vi "Test Preview Element.vi"() -> ()   [LabVIEW 2013]
uses:
  <vilib>/addons/_JKI Toolkits/Caraya/classes/Assert/Assert True.vi
  Circular Buffers/ByteFIFO/ByteFIFO.lvclass
  Circular Buffers/VariantBuffer/VariantBuffer.lvclass
  <vilib>/addons/_JKI Toolkits/Caraya/classes/Test/Test.lvclass
  <vilib>/addons/_JKI Toolkits/Caraya/classes/Assert/Assert.lvclass
panel:
  out "bytes 3":u8[](array[numeric]) format="%02x"
  out "bytes 2":u8[](array[numeric]) format="%02x"
  out "bytes":u8[](array[numeric]) format="%02x"
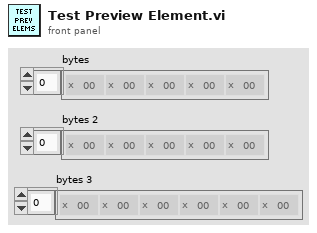
[diagram p1: front panel]
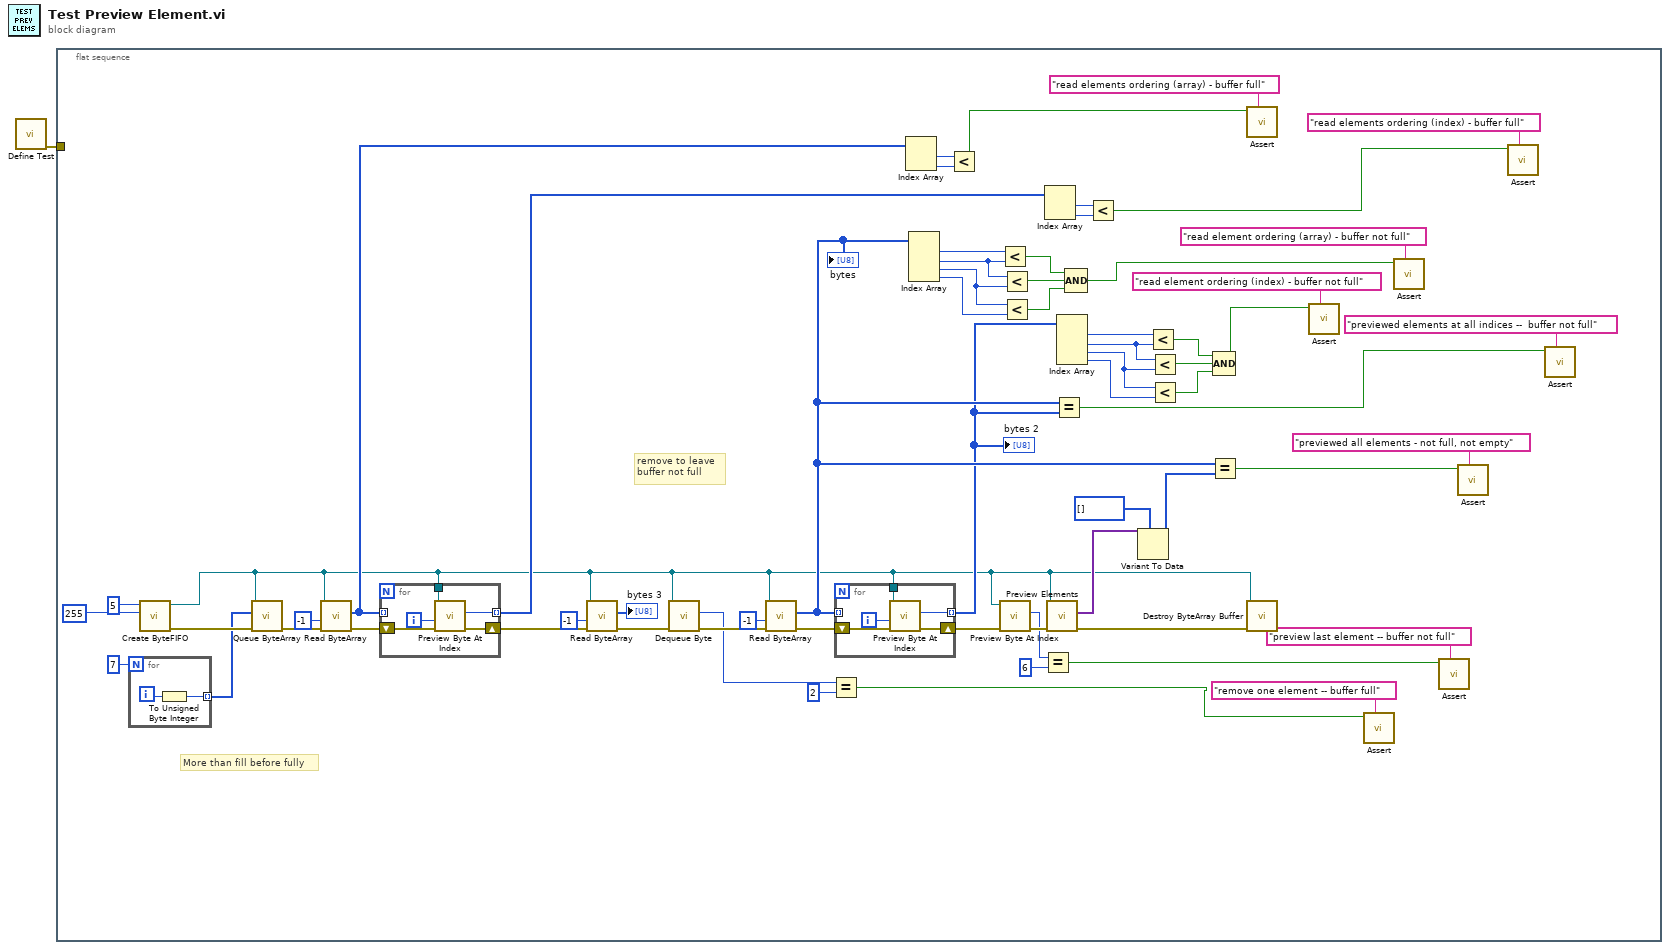
[diagram p0: block diagram]
diagram:
  n1 = call <vilib>:"Define Test.vi"() -> ("error out"=w1:errorcluster)  [unwired: 10 in, 1 out]
  n2 = flat-sequence {
    tunnel: w1 -> [_]
    frame #0 {
      # "remove to leave \nbuffer not full"
      # "More than fill before fully"
      n3 = for {
        N: 7 -> [_]
        tunnel: [w76] -> w61 mode=indexing
        i -> [w77]
        n4 = To Unsigned Byte Integer(number=w77) -> (unsigned 8bit integer=w76:u8)
      }
      n5 = call "Create ByteFIFO.vi"("default value"=u8 255, "bufSize"=5) -> ("error out"=w63:errorcluster, "Buffer"=w22:refnum<data-value>)  [unwired: 8 in]
      n6 = call "Queue ByteArray.vi"("error in"=w63, "bytes"=w61, "Buffer"=w22) -> ("error out"=w50:errorcluster)  [unwired: 6 in, 2 out]
      n7 = call "Read ByteArray.vi"("error in"=w50, "count (-1: all)"=-1, "Buffer"=w22) -> ("error out"=w47:errorcluster, "bytes"=w46:u8[])  [unwired: 6 in, 1 out]
      n8 = for {
        tunnel: w22 -> [w68]
        tunnel: [w67] -> w43 mode=indexing
        shift-right: [w66] -> w41
        shift-left: w47 -> [w70]
        tunnel: w46 -> [_] mode=indexing
        i -> [w69]
        n9 = call "Preview Byte At Index.vi"("error in (no error)"=w70, "index"=w69, "ByteFIFO"=w68) -> ("error out"=w66:errorcluster, "byte"=w67:u8)  [unwired: 5 in, 2 out]
      }
      n10 = call "Read ByteArray.vi"("error in"=w41, "count (-1: all)"=-1, "Buffer"=w22) -> ("error out"=w40:errorcluster, "bytes"=→"bytes 3":u8[])  [unwired: 6 in, 1 out]
      n11 = call "Dequeue Byte.vi"("error in"=w40, "Buffer"=w22) -> ("error out"=w60:errorcluster, "byte"=w24:u8)  [unwired: 5 in, 3 out]
      n12 = call "Read ByteArray.vi"("error in"=w60, "count (-1: all)"=-1, "Buffer"=w22) -> ("error out"=w59:errorcluster, "bytes"=w54:u8[])  [unwired: 6 in, 1 out]
      "bytes" <- w54
      n13 = Equal?(x=w24, y=u8 2) -> (x = y?=w3:bool)
      n14 = for {
        tunnel: w22 -> [w73]
        tunnel: w54 -> [_] mode=indexing
        tunnel: [w72] -> w25 mode=indexing
        shift-right: [w71] -> w21
        shift-left: w59 -> [w75]
        i -> [w74]
        n15 = call "Preview Byte At Index.vi"("error in (no error)"=w75, "index"=w74, "ByteFIFO"=w73) -> ("error out"=w71:errorcluster, "byte"=w72:u8)  [unwired: 5 in, 2 out]
      }
      "bytes 2" <- w25
      n16 = Index Array(array=w46) -> (element #1=w48:u8, element #2=w49:u8)  [unwired: 2 in]
      n17 = Index Array(array=w54) -> (element #1=w53:u8, element #2=w38:u8, element #3=w37:u8, element #4=w36:u8)  [unwired: 4 in]
      n18 = Less?(x=w48, y=w49) -> (x < y?=w16:bool)
      n19 = Less?(x=w53, y=w38) -> (x < y?=w33:bool)
      n20 = call "Preview Byte At Index.vi"("error in (no error)"=w21, "ByteFIFO"=w22) -> ("error out"=w20:errorcluster, "byte"=w18:u8)  [unwired: 6 in, 2 out]
      n21 = Less?(x=w38, y=w37) -> (x < y?=w35:bool)
      n22 = Less?(x=w37, y=w36) -> (x < y?=w34:bool)
      n23 = Equal?(x=w18, y=u8 6) -> (x = y?=w2:bool)
      n24 = Index Array(array=w43) -> (element #1=w45:u8, element #2=w44:u8)  [unwired: 2 in]
      n25 = call "Preview Elements.vi"("error in"=w20, "ByteBuffer in"=w22) -> ("error out"=w58:errorcluster, "elements"=w57:variant[])  [unwired: 7 in, 1 out]
      n26 = Equal?(x=w54, y=w25) -> (x = y?=w9:bool)
      n27 = Index Array(array=w25) -> (element #1=w26:u8, element #2=w27:u8, element #3=w28:u8, element #4=w29:u8)  [unwired: 4 in]
      n28 = Compound Arithmetic op=AND(w33, w35, w34) -> (w13:bool)
      n29 = Less?(x=w45, y=w44) -> (x < y?=w15:bool)
      n30 = Variant To Data(type=u8[] [], Variant=w57) -> (data=w55:u8[])  [unwired: 1 in, 1 out]
      n31 = Less?(x=w26, y=w27) -> (x < y?=w32:bool)
      n32 = Less?(x=w27, y=w28) -> (x < y?=w30:bool)
      n33 = Less?(x=w28, y=w29) -> (x < y?=w31:bool)
      n34 = Equal?(x=w54, y=w55) -> (x = y?=w7:bool)
      n35 = Compound Arithmetic op=AND(w32, w30, w31) -> (w11:bool)
      n36 = call-poly <vilib>:"Assert.vi"("Label"="read elements ordering (array) - buffer full", "True?"=w16) -> ()  [unwired: 8 in, 2 out]
      n37 = call "Destroy ByteArray Buffer.vi"("error in"=w58, "Buffer"=w22) -> ()  [unwired: 8 in, 2 out]
      n38 = call-poly <vilib>:"Assert.vi"("Label"="read element ordering (index) - buffer not full", "True?"=w11) -> ()  [unwired: 8 in, 2 out]
      n39 = call-poly <vilib>:"Assert.vi"("Label"="remove one element -- buffer full", "True?"=w3) -> ()  [unwired: 8 in, 2 out]
      n40 = call-poly <vilib>:"Assert.vi"("Label"="read element ordering (array) - buffer not full", "True?"=w13) -> ()  [unwired: 8 in, 2 out]
      n41 = call-poly <vilib>:"Assert.vi"("Label"="preview last element -- buffer not full", "True?"=w2) -> ()  [unwired: 8 in, 2 out]
      n42 = call-poly <vilib>:"Assert.vi"("Label"="previewed all elements - not full, not empty", "True?"=w7) -> ()  [unwired: 8 in, 2 out]
      n43 = call-poly <vilib>:"Assert.vi"("Label"="read elements ordering (index) - buffer full", "True?"=w15) -> ()  [unwired: 8 in, 2 out]
      n44 = call-poly <vilib>:"Assert.vi"("Label"="previewed elements at all indices --  buffer not full", "True?"=w9) -> ()  [unwired: 8 in, 2 out]
    }
  }
